vi "DC Bias State.vi"(6 "Curr Bias Monitor (F: Off)":bool, 7 "Volt Bias Monitor (F: Off)":bool, 8 "error in (no error)":errorcluster, 10 "State (F: Off)":bool, 11 "VISA resource name":refnum<visa-resource-name>) -> (0 "error out":errorcluster, 3 "VISA resource name out":refnum<visa-resource-name>)   [LabVIEW 2015, in "Agilent 428X Series.lvlib"]
doc: "This function sets the DC Bias, and DC Bias monitor function to ON or OFF."
uses:
  Agilent 428X Series.lvlib
panel:
  # "On\nOff"
  # "On\nOff"
  # "On\nOff"
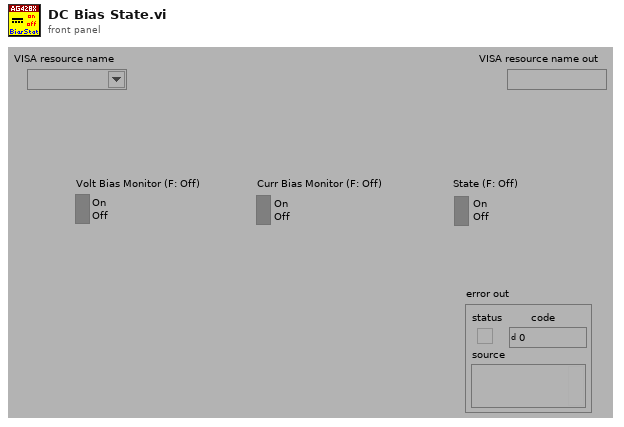
[diagram p1: front panel]
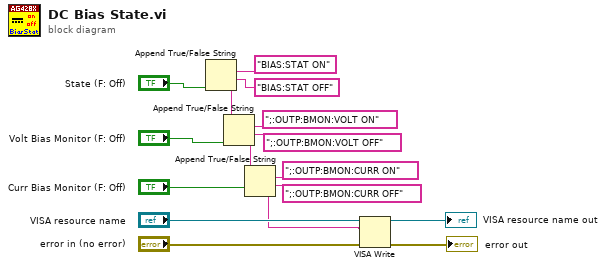
[diagram p0: block diagram]
diagram:
  n1 = Append True/False String(1:"State (F: Off)", 2:"BIAS:STAT OFF" ("false string"), 3:"BIAS:STAT ON" ("true string")) -> (0:w3:string)  [unwired: 1 in]
  n2 = Append True/False String(1:"Volt Bias Monitor (F: Off)", 2:";:OUTP:BMON:VOLT OFF" ("false string"), 3:";:OUTP:BMON:VOLT ON" ("true string"), 4:w3) -> (0:w2:string)
  n3 = Append True/False String(1:"Curr Bias Monitor (F: Off)", 2:";:OUTP:BMON:CURR OFF" ("false string"), 3:";:OUTP:BMON:CURR ON" ("true string"), 4:w2) -> (0:w1:string)
  n4 = VISA Write(VISA resource name="VISA resource name", write buffer=w1, error in (no error)="error in (no error)") -> (VISA resource name out=→"VISA resource name out":refnum<visa-resource-name>, error out=→"error out":errorcluster)  [unwired: 1 out]
